vi "has params.vi"(8 "error in (no error)":errorcluster, 11 "Request in":refnum<class "Request.lvclass">) -> (0 "error out":errorcluster, 2 "has params?":bool, 3 "Request out":refnum<class "Request.lvclass">)   [LabVIEW 2015, in "Request.lvclass"]
uses:
  Request.lvclass
  <vilib>/National Instruments/JSON Support for LabVIEW/JSON Types.ctl
  Request.lvclass/Request.ctl
  params/params.lvclass
  <vilib>/National Instruments/JSON Support for LabVIEW/JSON Data Classes/JSON Datatype/JSON Null.lvclass
  <vilib>/National Instruments/JSON Support for LabVIEW/LVJSON.lvlib
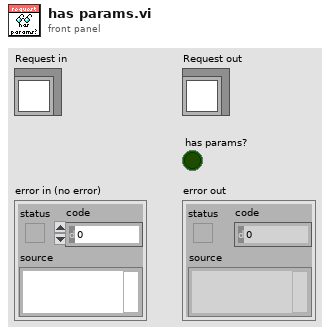
[diagram p1: front panel]
types:
  T1 = typedef "LVJSON.lvlib/JSON Types.ctl" = enum16{"String", "Numeric", "Boolean", "NULL", "Object", "Array"}
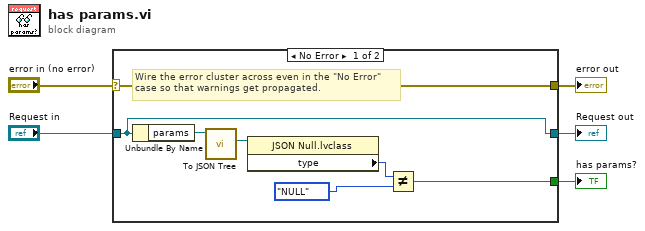
[diagram p0: block diagram]
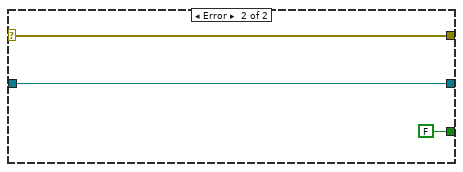
[diagram p2: hidden frame]
diagram:
  n1 = case shown="No Error" "error in (no error)" {
    selector: "error in (no error)" -> [w12 w15]
    tunnel: [w12 w15] -> w4
    tunnel: [w11 w14] -> w2
    tunnel: "Request in" -> [w11 w14]
    tunnel: [w10 FALSE] -> w1
    frame No Error {
      # "Wire the error cluster across even in the \"No Error\"\ncase so that warnings get propagated."
      n2 = Unbundle By Name(w11) -> ("params"=w9:refnum<class "params.lvclass">)
      n3 = call-dynamic "To JSON Tree.vi"("params in"=w9) -> ("JSON out"=w8:refnum<class "JSON Null.lvclass">)  [unwired: 8 in, 2 out]
      n4 = property class="JSON Null.lvclass"(reference=w8) -> ("type"=w7:T1)  [unwired: 1 in, 2 out]
      n5 = Not Equal?(x=w7, y=JSON_Types."NULL" ("type")) -> (x != y?=w10:bool)
    }
    frame Error {
    }
  }
  "error out" <- w4
  "Request out" <- w2
  "has params?" <- w1
